vi "sub_GSlam_calc-jacobian.vi"(11 "edge":T2) -> (2 "B":T1, 3 "A":T1)   [LabVIEW 2019]
uses:
  <vilib>/Analysis/Matrix/Datatypes/RealMatrix.ctl
  <vilib>/Analysis/Matrix/Numeric/Conversions/Array To Matrix - RA2.vi
  <vilib>/Analysis/Matrix/NI_Matrix.lvlib
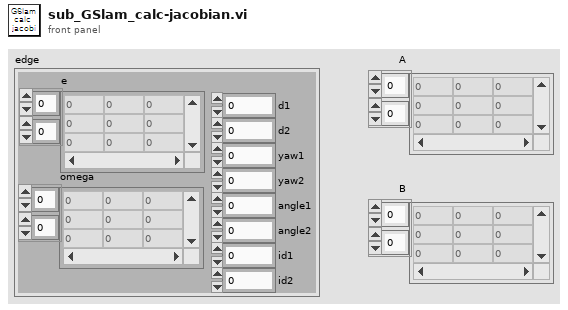
[diagram p1: front panel]
types:
  T1 = typedef "NI_Matrix.lvlib/RealMatrix.ctl" = dbl[][]
  T2 = cluster{"e":T1, "omega":T1, "d1":dbl, "d2":dbl, "yaw1":dbl, "yaw2":dbl, "angle1":dbl, "angle2":dbl, "id1":i32, "id2":i32}
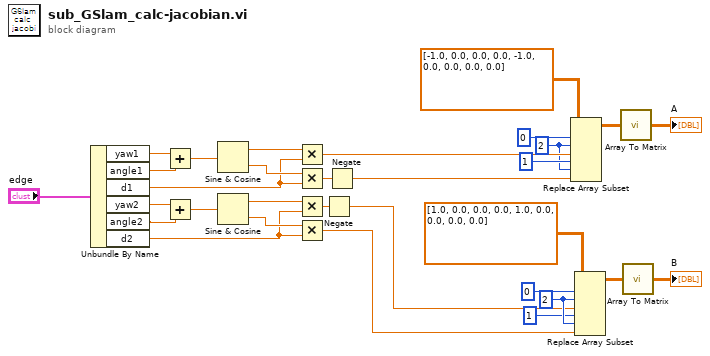
[diagram p0: block diagram]
diagram:
  w9 = 2 ("비활성화된 인덱스 (열)")
  w19 = 2 ("비활성화된 인덱스 (열)")
  n1 = Unbundle By Name("edge") -> ("yaw1"=w30:dbl, "angle1"=w29:dbl, "d1"=w25:dbl, "yaw2"=w16:dbl, "angle2"=w15:dbl, "d2"=w11:dbl)
  n2 = Add(x=w30, y=w29) -> (x+y=w28:dbl)
  n3 = Add(x=w16, y=w15) -> (x+y=w12:dbl)
  n4 = Sine & Cosine(0:w28) -> (1:w27:dbl, 2:w26:dbl)
  n5 = Sine & Cosine(0:w12) -> (1:w13:dbl, 2:w14:dbl)
  n6 = Multiply(x=w27, y=w25) -> (x*y=w23:dbl)
  n7 = Multiply(x=w26, y=w25) -> (x*y=w21:dbl)
  n8 = Multiply(x=w13, y=w11) -> (x*y=w5:dbl)
  n9 = Multiply(x=w14, y=w11) -> (x*y=w1:dbl)
  n10 = Negate(x=w5) -> (-x=w2:dbl)
  n11 = Negate(x=w21) -> (-x=w17:dbl)
  n12 = Replace Array Subset(array=dbl[][] [[-1.0, 0.0, 0.0], [0.0, -1.0, 0.0], [0.0, 0.0, 0.0]], new element #1=w23, index (row) #1=0 ("인덱스 (행)"), index (col) #1=w19, new element #2=w17, index (row) #2=1 ("인덱스 (행)"), index (col) #2=w19) -> (w18:dbl[][])
  n13 = Replace Array Subset(array=dbl[][] [[1.0, 0.0, 0.0], [0.0, 1.0, 0.0], [0.0, 0.0, 0.0]], new element #1=w2, index (row) #1=0 ("인덱스 (행)"), index (col) #1=w9, new element #2=w1, index (row) #2=1 ("인덱스 (행)"), index (col) #2=w9) -> (w10:dbl[][])
  n14 = call-poly <vilib>:"Array To Matrix.vi"("Real 2D Array"=w18) -> ("Real Matrix"=→"A":T1)
  n15 = call-poly <vilib>:"Array To Matrix.vi"("Real 2D Array"=w10) -> ("Real Matrix"=→"B":T1)
